vi "String cutter Temp and humidity subVI.vi"(0 "String":string) -> (1 "Temperature":dbl, 2 "Humidity":dbl)   [LabVIEW 2018]
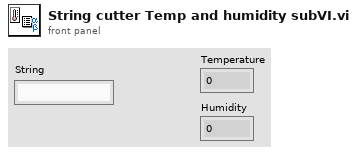
[diagram p1: front panel]
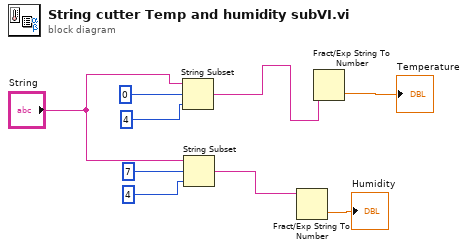
[diagram p0: block diagram]
diagram:
  n1 = String Subset(string="String", offset (0)=0, length (rest)=4) -> (substring=w4:string)
  n2 = String Subset(string="String", offset (0)=7, length (rest)=4) -> (substring=w5:string)
  n3 = Fract/Exp String To Number(string=w5) -> (number=→"Humidity":dbl)  [unwired: 3 in, 1 out]
  n4 = Fract/Exp String To Number(string=w4) -> (number=→"Temperature":dbl)  [unwired: 3 in, 1 out]
